vi "Controllers_PIDZPosition.vi"(0 "Task In":refnum<k21>, 1 "Beta":dbl=1.0, 2 "Alpha":dbl=nan format="%.2f", 5 "SP Femto":dbl=0.1, 7 "Piezo Offset In / V":dbl format="%.3g", 9 "Real time Femto / V":dbl=0.10000000000000014, 11 "Error In":errorcluster, 12 "DC Bias":dbl=0.2, 13 "PID gains":T1 {"derivative time (Td, min)" format="%.6f"; "integral time (Ti, min)" format="%.6f"; "proportional gain (Kc)" format="%.6f"}) -> (4 "Task Out":refnum<k21>, 6 "Stopped?":bool, 8 "Piezo Offset Out / V":dbl format="%.6g", 10 "Runtime / s":dbl, 15 "Error Out":errorcluster)   [LabVIEW 2022 SP3]
uses:
  <vilib>/DAQmx/write.llb/DAQmx Write (Analog 1D DBL NChan 1Samp).vi
  <vilib>/addons/control/pid/pid.llb/PID Advanced (DBL).vi
  <vilib>/DAQmx/miscellaneous.llb/DAQmx Fill In Error Info.vi
  <vilib>/addons/control/pid/NI_PID_pid.lvlib
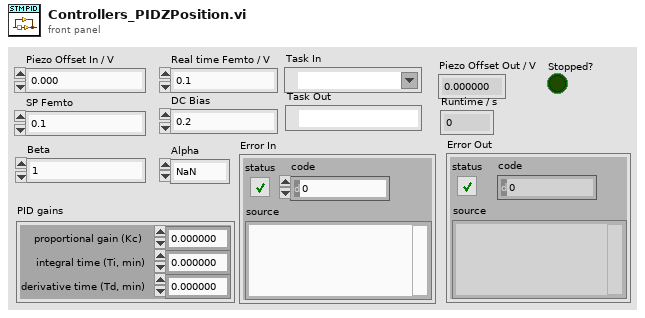
[diagram p1: front panel]
types:
  T1 = cluster{"proportional gain (Kc)":dbl, "integral time (Ti, min)":dbl, "derivative time (Td, min)":dbl}
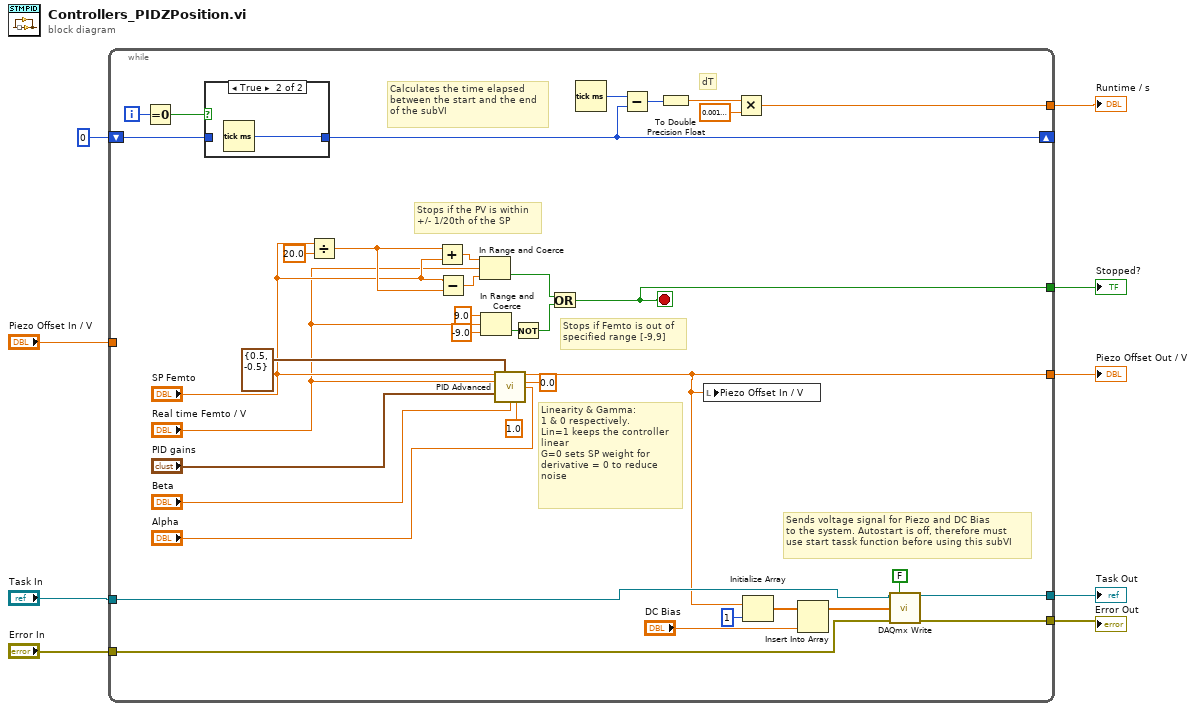
[diagram p0: block diagram]
diagram:
  n1 = while {
    tunnel: [w38] -> w9
    tunnel: "Task In" -> [w37]
    tunnel: [w36] -> w7
    tunnel: "Error In" -> [w35]
    shift-right: [w29] -> _
    shift-left: 0 -> [w30]
    tunnel: [w25] -> w4
    tunnel: [w12] -> w3
    tunnel: [w10] -> w2
    tunnel: "Piezo Offset In / V" -> [_]
    i -> [w31]
    stop <- w12 stop-if-true
    # "Stops if Femto is out of\nspecified range [-9,9]"
    # "Linearity & Gamma:\n1 & 0 respectively.\nLin=1 keeps the controller \nlinear\nG=0 sets SP weight for \nderivative = 0 to reduce\nnoise"
    # "Calculates the time elapsed\nbetween the start and the end\nof the subVI"
    # "Sends voltage signal for Piezo and DC Bias\nto the system. Autostart is off, therefore must\nuse start tassk function before using this subVI"
    # "Stops if the PV is within\n+/- 1/20th of the SP"
    # "dT"
    n2 = Equal To 0?(x=w31) -> (x = 0?=w13:bool)
    n3 = case shown="True" w13 {
      tunnel: [w47 w48] -> w29
      tunnel: w30 -> [w47 _]
      frame False {
      }
      frame True {
        n4 = Tick Count (ms)() -> (millisecond timer value=w48:u32)
      }
    }
    n5 = Divide(x="SP Femto", y=20.0) -> (x/y=w20:dbl)
    n6 = Add(x=w20, y="SP Femto") -> (x+y=w22:dbl)
    n7 = Subtract(x="SP Femto", y=w20) -> (x-y=w21:dbl)
    n8 = In Range and Coerce(upper limit=w22, x="Real time Femto / V", lower limit=w21) -> (In Range?=w15:bool)  [unwired: 1 out]
    n9 = In Range and Coerce(upper limit=9.0, x="Real time Femto / V", lower limit=-9.0) -> (In Range?=w19:bool)  [unwired: 1 out]
    n10 = call-poly <vilib>:"PID Advanced.vi"("setpoint"="SP Femto", "output range"=cluster{"output high":dbl, "output low":dbl} {"output high"=0.5, "output low"=-0.5}, "process variable"="Real time Femto / V", "gamma"=0.0, "alpha"="Alpha", "PID gains"="PID gains", "beta"="Beta", "linearity"=1.0) -> ("output"=w10:dbl)  [unwired: 6 in, 1 out]
    n11 = Not(x=w19) -> (.not. x?=w16:bool)
    n12 = Or(x=w15, y=w16) -> (x .or. y?=w12:bool)
    n13 = Tick Count (ms)() -> (millisecond timer value=w32:u32)
    n14 = Subtract(x=w32, y=w29) -> (x-y=w26:u32)
    n15 = To Double Precision Float(number=w26) -> (double precision float=w28:dbl)
    n16 = local write "Piezo Offset In / V"(w10) -> ()
    n17 = Multiply(x=w28, y=0.0010000000474974513) -> (x*y=w25:dbl)
    n18 = Initialize Array(w10, 1 ("dimension size")) -> (w41:dbl[])
    n19 = Insert Into Array(array=w41, new element="DC Bias") -> (w40:dbl[])  [unwired: 1 in]
    n20 = call-poly <vilib>:"DAQmx Write.vi"("task/channels in"=w37, "auto start"=FALSE, "data"=w40, "error in"=w35) -> ("task out"=w38:refnum<k21>, "error out"=w36:errorcluster)  [unwired: 9 in, 1 out]
  }
  "Task Out" <- w9
  "Error Out" <- w7
  "Runtime / s" <- w4
  "Stopped?" <- w3
  "Piezo Offset Out / V" <- w2
